vi "itc_collect_pixelEvents.vi"() -> ()   [LabVIEW 2016]
uses:
  <vilib>/rvi/Emulation/niFpgaEmulationIsFPGAContextNoSignature.vi
  <vilib>/rvi/Emulation/niFpgaSctlEmulationGetInTimedLoop.vi
  <vilib>/rvi/errors/niFpgaSetErrorForExecOnDevCompSimple.vi
  <vilib>/rvi/eio/common/nirviEmuReportErrorAndStop.vi
  <vilib>/rvi/DataTransferAndStorage/Container/Common/niFpgaContainerGetUniqueNameForEmu.vi
  <vilib>/rvi/FIFO/Fifo_Resource/nirvififoEmulationSetSize.vi
  <vilib>/rvi/FIFO/Fifo_Resource/nirviFifoEmulationQueueMgr.vi
  <instcachedir>/1/nirviFifoEmulationQueueMgr_E5CAEC123FF24DC58D834DCA3CDAA9B5.lvgen/nirviFifoEmulationQueueMgr_E5CAEC123FF24DC58D834DCA3CDAA9B5_000.vi
  <vilib>/Utility/error.llb/Clear Errors.vi
  <vilib>/rvi/FIFO/Fifo_Resource/nirvififoEmulationCreateLock.vi
  <vilib>/rvi/Emulation/niFpgaProcessEmulError.vi
  <vilib>/rvi/FIFO/Fifo_Resource/nirvififoEmulationObtainLock.vi
  <vilib>/rvi/FIFO/Fifo_Resource/nirvififoEmulationReleaseLock.vi
  <vilib>/rvi/occurrence/nirviWaitOnOccurrenceBase.vi
  <vilib>/rvi/errors/nirviReportUnexpectedCaseInternalError.vi
  <vilib>/rvi/errors/nirviReportUnexpectedCaseInternalError (U32).vi
  <vilib>/rvi/eio/common/nirviEmuTemplateMethod_errors.vi
  <vilib>/rvi/DataTransferAndStorage/Container/XNode/niFpgaContainer.xnode
  <vilib>/rvi/FIFO/Fifo_Resource/nirvififoEmulationRead.vi
  <vilib>/eio/EIONode/EIONode.xnode
panel:
  out "se.s.ticksPerPixel":u32
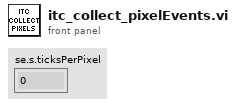
[diagram p1: front panel]
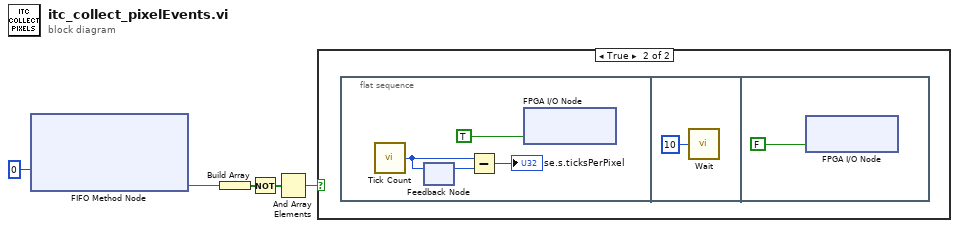
[diagram p0: block diagram]
diagram:
  n1 = xnode ("FIFO Method Node")("Timeout"=0) -> ("Timed Out?"=w4:bool)  [unwired: 1 in, 2 out]
  n2 = Build Array(w4) -> (w3:bool[])
  n3 = Not(x=w3) -> (.not. x?=w2:bool[])
  n4 = And Array Elements(Boolean array=w2) -> (logical AND=w5:bool)
  n5 = case shown="True" w5 {
    frame False {
    }
    frame True {
      n6 = flat-sequence {
        frame #0 {
          n7 = call "Tick Count"() -> ("Tick Count(Ticks)"=w7:u32)
          n8 = feedback #1() -> (w8:u32)  [unwired: 1 in]
          n9 = feedback-in #1(w7) -> ()
          n10 = Subtract(x=w7, y=w8) -> (x-y=→"se.s.ticksPerPixel":u32)
          n11 = xnode "FPGA I/O Node"("pixelSync"=TRUE) -> ()  [unwired: 1 in, 1 out]
        }
        frame #1 {
          n12 = call "Wait"("Count(Ticks)"=u32 10) -> ()  [unwired: 1 out]
        }
        frame #2 {
          n13 = xnode "FPGA I/O Node"("pixelSync"=FALSE) -> ()  [unwired: 1 in, 1 out]
        }
      }
    }
  }
